vi "Nod_Head.vi"(0 "error in":errorcluster, 2 "State":bool=TRUE, 3 "node":string) -> (1 "error out":errorcluster)   [LabVIEW 2013]
doc: "This will nod the head."
uses:
  ROS/MessageBuilding/Primitives/subs/boolScalar.vi
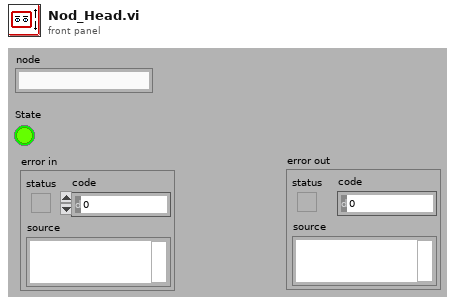
[diagram p1: front panel]
types:
  T1 = typedef "_ROSControl.ctl" = cluster{"topic port":u16, "Node":string, "topic":string, "type":string, "node port":u32, "error ":errorcluster, "Direction":T2, "APIs":string[]}
  T2 = typedef "_ROSDirection.ctl" = enum16{"Node", "Publisher", "Subscriber", "Service Client"}
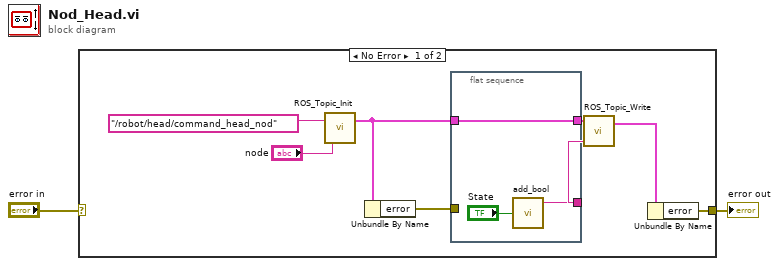
[diagram p0: block diagram]
diagram:
  n1 = case shown="No Error" "error in" {
    selector: "error in" -> [_ w14]
    tunnel: [w8 w14] -> w2
    frame No Error {
      n2 = call "ROS_Topic_Init.vi"("node"="node", "topic"="/robot/head/command_head_nod") -> ("ROS out"=w4:T1)  [unwired: 1 in]
      n3 = Unbundle By Name(w4) -> ("error"=w3:errorcluster)
      n4 = flat-sequence {
        tunnel: [w13] -> w6
        tunnel: w4 -> [w11]
        tunnel: [w11] -> w5
        tunnel: w3 -> [_]
        frame #0 {
          n5 = call-poly "add_bool.vi"("Boolean"="State") -> ("msg out"=w13:string)  [unwired: 4 in]
        }
      }
      n6 = call "ROS_Topic_Write.vi"("Msg in"=w6, "ROS in"=w5) -> ("ROS out"=w9:T1)  [unwired: 2 in]
      n7 = Unbundle By Name(w9) -> ("error"=w8:errorcluster)
    }
    frame Error {
    }
  }
  "error out" <- w2
